vi "SE FP hindbrain THINK.vi"(2 "error in":errorcluster, 3 "BLUE LED":bool=TRUE, 4 "GREEN LED":bool=TRUE, 5 "RED LED":bool=TRUE) -> (0 "error out":errorcluster, 1 "LED array":bool[](array[boolean]))   [LabVIEW 2014]
doc: "This vi is the THINK portion of the Hindbrain...at present it has not function and is a place holder for later development."
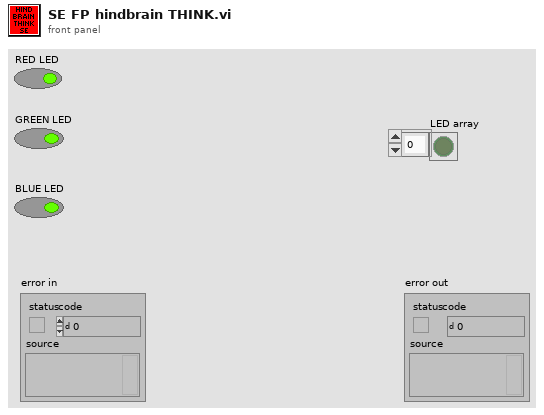
[diagram p1: front panel]
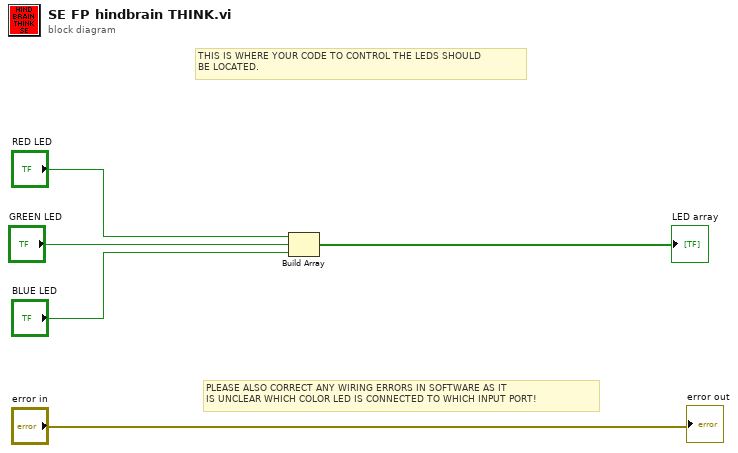
[diagram p0: block diagram]
diagram:
  # "PLEASE ALSO CORRECT ANY WIRING ERRORS IN SOFTWARE AS IT\nIS UNCLEAR WHICH COLOR LED IS CONNECTED TO WHICH INPUT PORT!"
  # "THIS IS WHERE YOUR CODE TO CONTROL THE LEDS SHOULD\nBE LOCATED."
  n1 = Build Array("RED LED", "GREEN LED", "BLUE LED") -> (→"LED array":bool[])
  "error out" <- "error in"
